vi "FTW-SQLite-PrepareStatement.vi"(0 "SQLite Connector":refnum<class "FTW-SQLite-Connector.lvclass">, 5 "SQL Statement":string, 11 "error in":errorcluster) -> (4 "SQLite Connector out":refnum<class "FTW-SQLite-Connector.lvclass">, 6 "Prepared Statements":i64[](array[numeric]) format="0x%016x", 8 "Time to Compile SQL":dbl format="%.6fsec", 15 "error out":errorcluster)   [LabVIEW 2012, in "FTW-SQLite-Connector.lvclass"]
uses:
  FTW-SQLite-Connector.lvclass
  FTW-SQLite-Connector.lvclass/FTW-SQLite-Connector.ctl
panel:
  # "Inputs"
  # "Outputs"
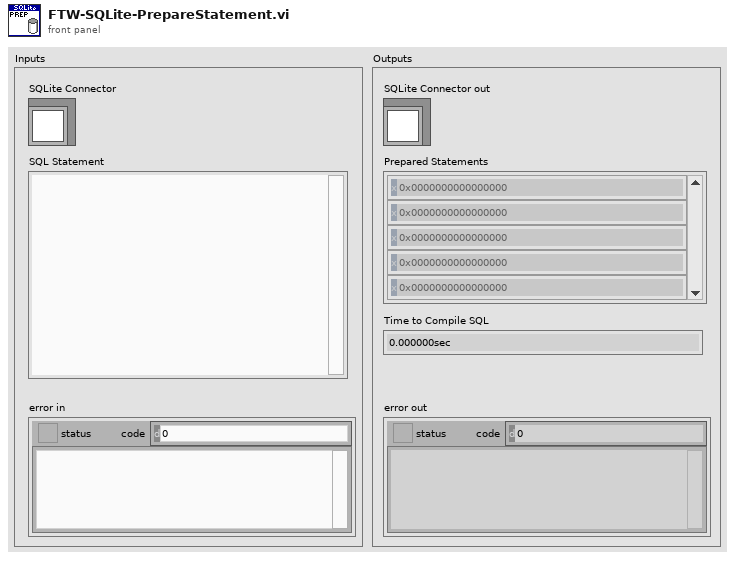
[diagram p1: front panel]
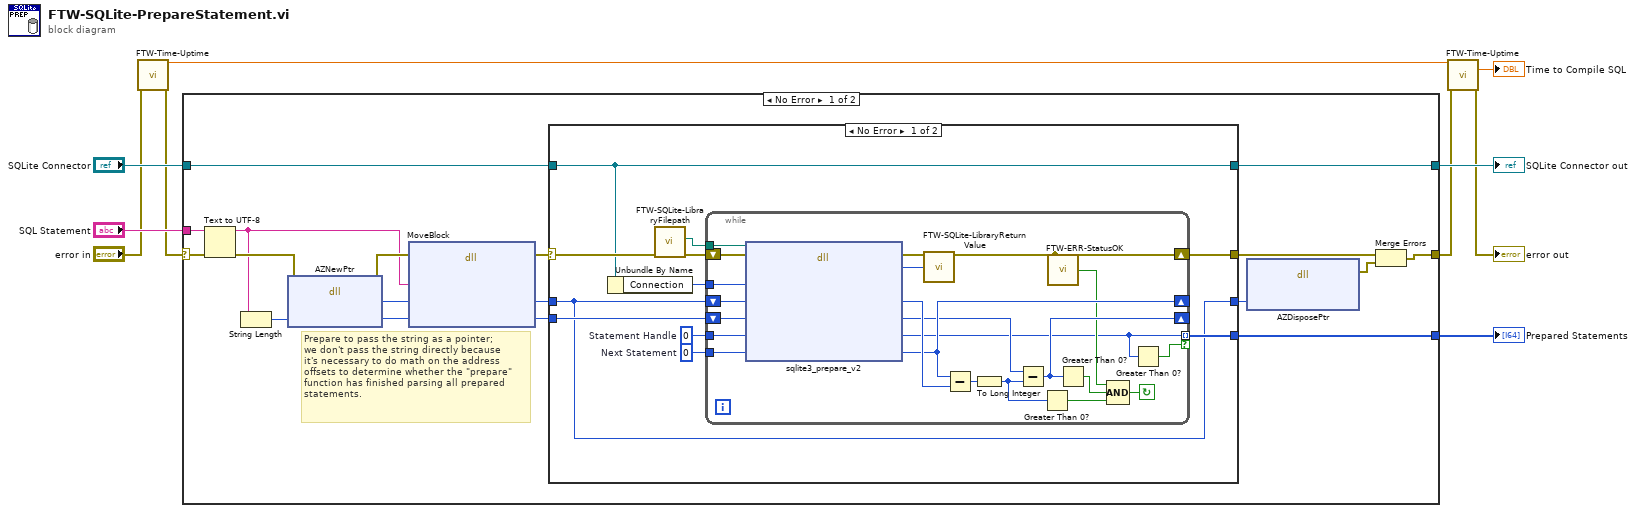
[diagram p0: block diagram]
diagram:
  n1 = call "FTW-Time-Uptime.vi"("error in"="error in") -> ("Current Uptime"=w2:dbl, "error out"=w5:errorcluster)  [unwired: 12 in, 1 out]
  n2 = case shown="No Error" w5 {
    selector: w5 -> [w14 w65]
    tunnel: "SQLite Connector" -> [w28 w66]
    tunnel: [w27 w66] -> w9
    tunnel: "SQL Statement" -> [w26 _]
    tunnel: [w16 w65] -> w3
    tunnel: [w15 _] -> w7
    frame No Error {
      # "Prepare to pass the string as a pointer;\nwe don't pass the string directly because\nit's necessary to do math on the address\noffsets to determine whether the \"prepare\"\nfunction has finished parsing all prepared\nstatements."
      n3 = Text to UTF-8(8:w14, 11:w26) -> (0:w21:errorcluster, 3:w20:string)
      n4 = String Length(string=w20) -> (length=w25:i32)
      n5 = dll-call lib="LabVIEW" fn="AZNewPtr"(error in=w21, "Data Size"=w25) -> (error out=w24:errorcluster, "New Pointer"=w23:i64, "Data Size"=w22:i32)  [unwired: 2 in, 1 out]
      n6 = dll-call lib="LabVIEW" fn="MoveBlock"(error in=w24, "Source String"=w20, "Pointer to Destination"=w23, "String Length"=w22) -> (error out=w11:errorcluster, "Pointer to Destination"=w18:i64, "String Length"=w19:i32)  [unwired: 4 in, 1 out]
      n7 = case shown="No Error" w11 {
        selector: w11 -> [w31 w63]
        tunnel: w28 -> [w29 w64]
        tunnel: [w29 w64] -> w27
        tunnel: w19 -> [w39 _]
        tunnel: w18 -> [w32 w62]
        tunnel: [w38 w63] -> w17
        tunnel: [w37 _] -> w15
        tunnel: [w32 w62] -> w13
        frame No Error {
          w35 = i64 0  # Next Statement
          w36 = i64 0  # Statement Handle
          n8 = Unbundle By Name(w29) -> ("Connection"=w30:u64)
          n9 = call "FTW-SQLite-LibraryFilepath.vi"("error in"=w31) -> ("error out"=w34:errorcluster, "SQLite Library Filepath"=w33:path)  [unwired: 8 in, 1 out]
          n10 = while {
            tunnel: [w41] -> w37 mode=indexing if=w55
            shift-right: [w54] -> _
            shift-left: w32 -> [w57]
            shift-right: [w48] -> _
            shift-left: w39 -> [w56]
            tunnel: w36 -> [w46]
            tunnel: w35 -> [w45]
            tunnel: w33 -> [w44]
            shift-right: [w40] -> w38
            shift-left: w34 -> [w43]
            tunnel: w30 -> [w58]
            stop <- w51 continue-if-true
            n11 = dll-call lib="?" fn="sqlite3_prepare_v2"(path in=w44, error in=w43, "Connection Handle"=w58, "SQL Statement Pointer"=w57, "Statement Length"=w56, "Prepared Statement Pointer"=w46, "Next Statement Pointer"=w45) -> (error out=w60:errorcluster, "Return Value"=w59:i32, "SQL Statement Pointer"=w61:i64, "Statement Length"=w50:i32, "Prepared Statement Pointer"=w41:i64, "Next Statement Pointer"=w54:i64)  [unwired: 2 in, 1 out]
            n12 = call "FTW-SQLite-LibraryReturnValue.vi"("error in"=w60, "Return Value"=w59) -> ("error out"=w40:errorcluster)  [unwired: 13 in]
            n13 = Subtract(x=w54, y=w61) -> (x-y=w49:i64)
            n14 = To Long Integer(number=w49) -> (32bit integer=w47:i32)
            n15 = Subtract(x=w50, y=w47) -> (x-y=w48:i32)
            n16 = Greater Than 0?(x=w47) -> (x > 0?=w53:bool)
            n17 = call "FTW-ERR-StatusOK.vi"("error to check"=w40) -> ("Status OK?"=w42:bool)
            n18 = Greater Than 0?(x=w48) -> (x > 0?=w52:bool)
            n19 = Compound Arithmetic op=AND(w42, w52, w53) -> (w51:bool)
            n20 = Greater Than 0?(x=w41) -> (x > 0?=w55:bool)
          }
        }
        frame Error {
        }
      }
      n21 = dll-call lib="LabVIEW" fn="AZDisposePtr"("Pointer Address"=w13) -> (error out=w12:errorcluster)  [unwired: 5 in, 1 out]
      n22 = Merge Errors(w17, w12) -> (w16:errorcluster)
    }
    frame Error {
    }
  }
  "SQLite Connector out" <- w9
  "Prepared Statements" <- w7
  n23 = call "FTW-Time-Uptime.vi"("Previous Uptime"=w2, "error in"=w3) -> ("Elapsed Time"=→"Time to Compile SQL":dbl, "error out"=→"error out":errorcluster)  [unwired: 11 in, 1 out]
